vi "Set Core APIs.vi"(8 "error in (no error)":errorcluster, 10 "Core APIs":T1, 11 "Task in":refnum<class "Task.lvclass">) -> (0 "error out":errorcluster, 3 "Task out":refnum<class "Task.lvclass">)   [LabVIEW 2020, in "Volatus.lvlib" / "Task.lvclass"]
uses:
  Task.lvclass
  Core APIs.ctl
  VolatusAPI/VolatusAPI.lvclass
  Event API/EventAPI.lvclass
  ConfigAPI/ConfigAPI.lvclass
  Task.lvclass/Task.ctl
  Volatus.lvlib
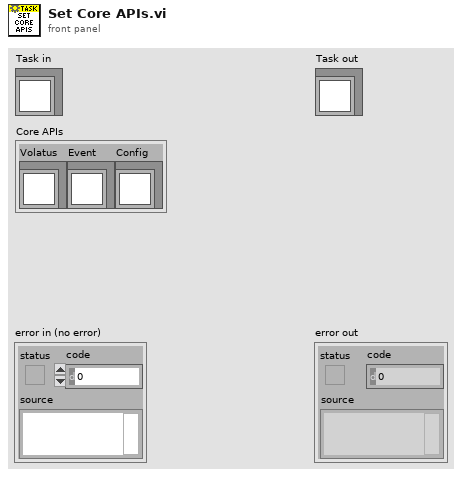
[diagram p1: front panel]
types:
  T1 = typedef "Volatus.lvlib/Core APIs.ctl" = cluster{"Volatus":refnum<class "VolatusAPI.lvclass">, "Event":refnum<class "EventAPI.lvclass">, "Config":refnum<class "ConfigAPI.lvclass">}
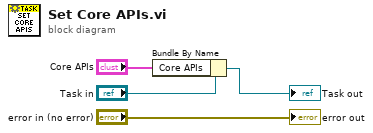
[diagram p0: block diagram]
diagram:
  n1 = Bundle By Name(cluster="Task in", "Core APIs"="Core APIs") -> (→"Task out":refnum<class "Task.lvclass">)
  "error out" <- "error in (no error)"
